vi "Destroy Data Channels.vi"(8 "error in":errorcluster, 11 "Node in":refnum<class "ThermotronDriver.lvclass">) -> (0 "error out":errorcluster, 3 "Node out":refnum<class "ThermotronDriver.lvclass">)   [LabVIEW 2023, in "ThermotronDriver.lvlib" / "ThermotronDriver.lvclass"]
uses:
  ThermotronDriver.lvclass
  ThermotronDriver.lvclass/ThermotronDriver.ctl
  <vilib>/ADAS Replay HIL/AdasHilServices/AdasHilChannelServices.lvlib
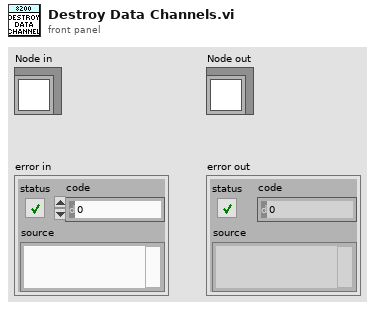
[diagram p1: front panel]
types:
  T1 = cluster{"Counter.AV":refnum<k21>, "Air_Temperature.AV":refnum<k21>, "Initialized.STS":refnum<k21>, "On_Off.STS":refnum<k21>}
  T2 = cluster{"Air_Temperature.SP":refnum<k21>, "On_Off.ACT":refnum<k21>}
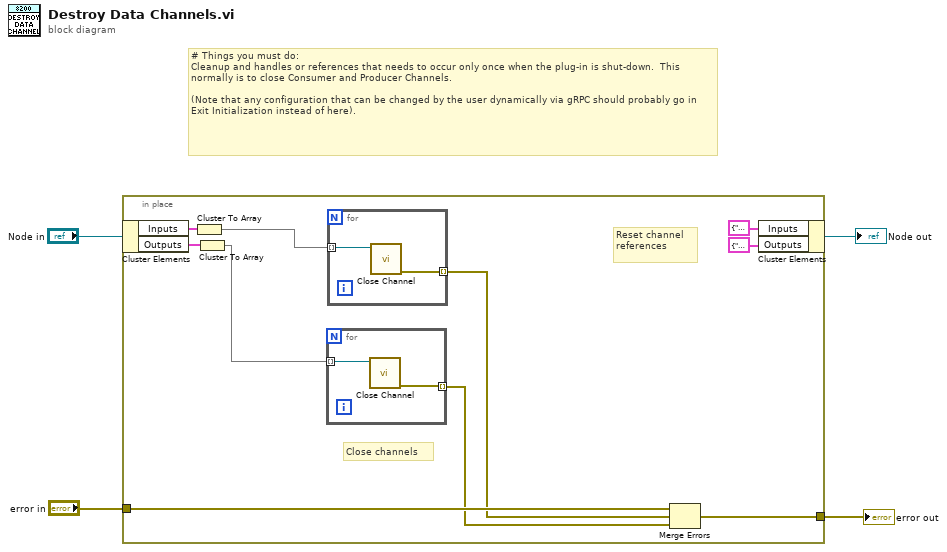
[diagram p0: block diagram]
diagram:
  # "# Things you must do:\nCleanup and handles or references that needs to occur only once when the plug-in is shut-down.  This normally is to close Consumer and Producer Channels.   \n\n(Note that any configuration that can be changed by the user dynamically via gRPC should probably go in Exit Initialization instead of here)."
  n1 = in-place {
    in-place-border: [w13] -> w1
    in-place-border: "error in" -> [w14]
    # "Reset channel\nreferences"
    # "Close channels"
    n2 = in-place-cluster #1("Node in") -> ("Inputs"=w12:T2, "Outputs"=w10:T1)
    n3 = Cluster To Array(cluster=w12) -> (array=w11:refnum<k21>[])
    n4 = Cluster To Array(cluster=w10) -> (array=w9:refnum<k21>[])
    n5 = for {
      tunnel: w9 -> [w16] mode=indexing
      tunnel: [w15] -> w7 mode=indexing
      n6 = call <vilib>:"Close Channel.vi"("ADAS HIL Channel"=w16) -> ("error out"=w15:errorcluster)  [unwired: 10 in]
    }
    n7 = for {
      tunnel: w11 -> [w18] mode=indexing
      tunnel: [w17] -> w8 mode=indexing
      n8 = call <vilib>:"Close Channel.vi"("ADAS HIL Channel"=w18) -> ("error out"=w17:errorcluster)  [unwired: 10 in]
    }
    n9 = Merge Errors(w14, w8, w7) -> (w13:errorcluster)
    n10 = in-place-cluster #1("Inputs"=T2 {"Air_Temperature.SP"="", "On_Off.ACT"=""}, "Outputs"=T1 {"Counter.AV"="", "Air_Temperature.AV"="", "Initialized.STS"="", "On_Off.STS"=""}) -> (→"Node out":refnum<class "ThermotronDriver.lvclass">)
  }
  "error out" <- w1
